vi "ClearFP.vi"(8 "error in":errorcluster, 11 "reference":refnum<vi>) -> (0 "error out":errorcluster, 3 "reference out":refnum<vi>)   [LabVIEW 2013]
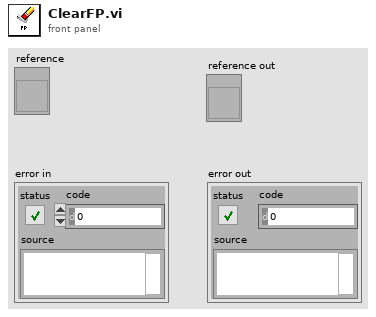
[diagram p1: front panel]
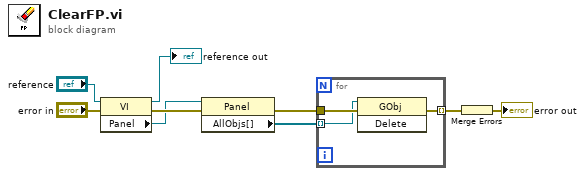
[diagram p0: block diagram]
diagram:
  n1 = property class="VI"(reference="reference", error in="error in") -> (reference out=→"reference out":refnum<vi>, error out=w9:errorcluster, "Panel"=w8:refnum<vi>)
  n2 = property class="Panel"(reference=w8, error in=w9) -> (error out=w7:errorcluster, "AllObjs[]"=w6:refnum<vi>[])  [unwired: 1 out]
  n3 = for {
    tunnel: w7 -> [w12]
    tunnel: w6 -> [w11] mode=indexing
    tunnel: [w10] -> w5 mode=indexing
    n4 = invoke class="GObj" method="Delete"(reference=w11, error in=w12) -> (error out=w10:errorcluster)  [unwired: 1 in, 2 out]
  }
  n5 = Merge Errors(w5) -> (→"error out":errorcluster)
